vi "RPC Method GreeterService GetFeature.vi"(3 "error in (no error)":errorcluster, 4 "gRPCid in":T1, 5 "DNL_LabVIEW Object in":refnum<class "GreeterServiceImpl.lvclass">) -> (0 "error out":errorcluster, 1 "gRPCid out":T1, 2 "DNL_LabVIEW Object out":refnum<class "GreeterServiceImpl.lvclass">)   [LabVIEW 2019, in "UserCode_impl_server.lvlib" / "GreeterServiceImpl.lvclass"]
uses:
  GreeterServiceImpl.lvclass
  <vilib>/gRPC/LabVIEW gRPC Library/Shared/grpcId.ctl
  Generated_stub_server/RPC Messages/Greeter_res.ctl
  Generated_stub_server/RPC Messages/Greeter_res_res_oneof/Greeter_res_res_oneof.lvclass
  Generated_stub_server/RPC Messages/Greeter_req_req_oneof/Greeter_req_req_oneof.lvclass/Greeter_req_req_oneof.ctl
  Generated_stub_server/RPC Messages/Greeter_res_res_oneof/Greeter_res_res_oneof.lvclass/Greeter_res_res_oneof.ctl
  Generated_stub_server/Generated_stub_server.lvlib
  Generated_stub_server/RPC Messages/Greeter_req_req_oneof/Greeter_req_req_oneof.lvclass
  Generated_stub_server/RPC Service/GreeterServiceStub/GreeterServiceStub.lvclass
  <vilib>/gRPC/LabVIEW gRPC Library/grpc-lvsupport-release.lvlib
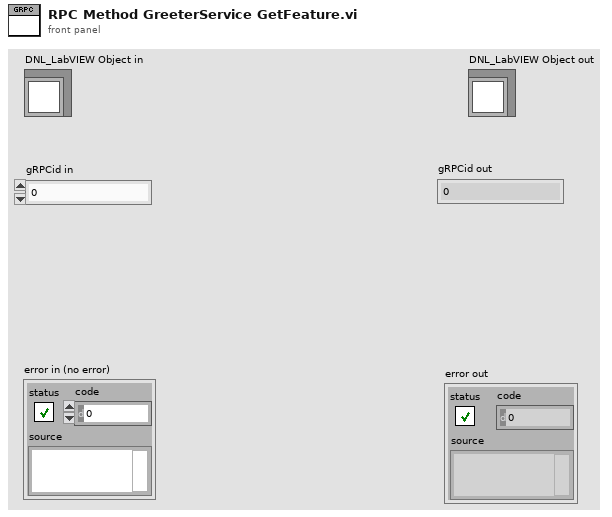
[diagram p1: front panel]
types:
  T1 = typedef "grpc-lvsupport-release.lvlib/grpcId.ctl" = u64
  T2 = typedef "Generated_stub_server.lvlib/Greeter_res.ctl" = cluster{"res_latitude":i32, "Greeter_res_res_oneof":refnum<class "Greeter_res_res_oneof.lvclass">}
  T3 = typedef "Generated_stub_server.lvlib/Greeter_req.ctl" = cluster{"req_latitude":i32, "Greeter_req_req_oneof":refnum<class "Greeter_req_req_oneof.lvclass">}
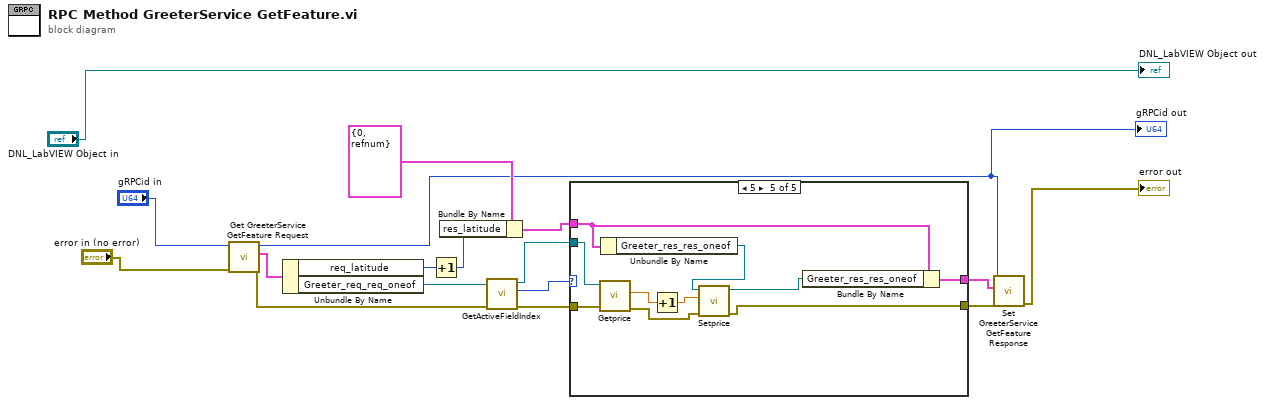
[diagram p0: block diagram]
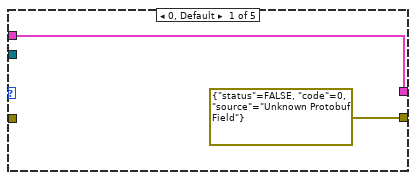
[diagram p2: hidden frame]
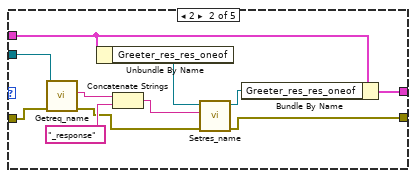
[diagram p3: hidden frame]
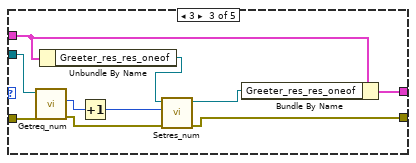
[diagram p4: hidden frame]
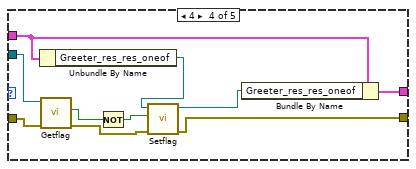
[diagram p5: hidden frame]
diagram:
  n1 = call "Get GreeterService GetFeature Request.vi"("error in (no error)"="error in (no error)", "gRPCid"="gRPCid in") -> ("error out"=w15:errorcluster, "Message Data"=w17:T3, "gRPCid out"=w2:T1)  [unwired: 7 in]
  "gRPCid out" <- w2
  n2 = Unbundle By Name(w17) -> ("req_latitude"=w11:i32, "Greeter_req_req_oneof"=w16:refnum<class "Greeter_req_req_oneof.lvclass">)
  n3 = Increment(x=w11) -> (x+1=w10:i32)
  n4 = Bundle By Name(cluster=T2 {"res_latitude"=0, "Greeter_res_res_oneof"=refnum} ("Greeter_res"), "res_latitude"=w10) -> (w9:T2)
  n5 = call "GetActiveFieldIndex.vi"("error in (no error)"=w15, "OneOfTemplate in"=w16) -> ("error out"=w12:errorcluster, "Active Field Index"=w14:i32, "OneOfTemplate out"=w13:refnum<class "Greeter_req_req_oneof.lvclass">)  [unwired: 7 in]
  n6 = case shown="5" w14 {
    tunnel: w13 -> [_ w30 w38 w48 w59]
    tunnel: w12 -> [_ w29 w37 w47 w58]
    tunnel: w9 -> [w18 w23 w40 w50 w60]
    tunnel: [w18 w21 w39 w49 w52] -> w7
    tunnel: [errorcluster {"status"=FALSE, "code"=0, "source"="Unknown Protobuf Field"} ("error out") w20 w32 w41 w51] -> w8
    frame 0, Default {
    }
    frame 2 {
      n7 = call "Getreq_name.vi"("error in (no error)"=w29, "OneOfTemplate in"=w30) -> ("error out"=w24:errorcluster, "Get_Val"=w28:string)  [unwired: 7 in, 1 out]
      n8 = Unbundle By Name(w23) -> ("Greeter_res_res_oneof"=w26:refnum<class "Greeter_res_res_oneof.lvclass">)
      n9 = Concatenate Strings(w28, "_response" ("string")) -> (w25:string)
      n10 = call "Setres_name.vi"("error in (no error)"=w24, "Set_Val"=w25, "OneOfTemplate in"=w26) -> ("error out"=w20:errorcluster, "OneOfTemplate out"=w22:refnum<class "Greeter_res_res_oneof.lvclass">)  [unwired: 7 in]
      n11 = Bundle By Name(cluster=w23, "Greeter_res_res_oneof"=w22) -> (w21:T2)
    }
    frame 3 {
      n12 = call "Getreq_num.vi"("error in (no error)"=w37, "OneOfTemplate in"=w38) -> ("error out"=w31:errorcluster, "Get_Val"=w36:i32)  [unwired: 7 in, 1 out]
      n13 = Unbundle By Name(w40) -> ("Greeter_res_res_oneof"=w34:refnum<class "Greeter_res_res_oneof.lvclass">)
      n14 = Increment(x=w36) -> (x+1=w35:i32)
      n15 = call "Setres_num.vi"("error in (no error)"=w31, "Set_Val"=w35, "OneOfTemplate in"=w34) -> ("error out"=w32:errorcluster, "OneOfTemplate out"=w33:refnum<class "Greeter_res_res_oneof.lvclass">)  [unwired: 7 in]
      n16 = Bundle By Name(cluster=w40, "Greeter_res_res_oneof"=w33) -> (w39:T2)
    }
    frame 4 {
      n17 = Unbundle By Name(w50) -> ("Greeter_res_res_oneof"=w44:refnum<class "Greeter_res_res_oneof.lvclass">)
      n18 = call "Getflag.vi"("error in (no error)"=w47, "OneOfTemplate in"=w48) -> ("error out"=w43:errorcluster, "Get_Val"=w46:bool)  [unwired: 7 in, 1 out]
      n19 = Not(x=w46) -> (.not. x?=w45:bool)
      n20 = call "Setflag.vi"("error in (no error)"=w43, "Set_Val"=w45, "OneOfTemplate in"=w44) -> ("error out"=w41:errorcluster, "OneOfTemplate out"=w42:refnum<class "Greeter_res_res_oneof.lvclass">)  [unwired: 7 in]
      n21 = Bundle By Name(cluster=w50, "Greeter_res_res_oneof"=w42) -> (w49:T2)
    }
    frame 5 {
      n22 = call "Getprice.vi"("error in (no error)"=w58, "OneOfTemplate in"=w59) -> ("error out"=w54:errorcluster, "Get_Val"=w56:sgl)  [unwired: 7 in, 1 out]
      n23 = Unbundle By Name(w60) -> ("Greeter_res_res_oneof"=w55:refnum<class "Greeter_res_res_oneof.lvclass">)
      n24 = Increment(x=w56) -> (x+1=w57:sgl)
      n25 = call "Setprice.vi"("error in (no error)"=w54, "Set_Val"=w57, "OneOfTemplate in"=w55) -> ("error out"=w51:errorcluster, "OneOfTemplate out"=w53:refnum<class "Greeter_res_res_oneof.lvclass">)  [unwired: 7 in]
      n26 = Bundle By Name(cluster=w60, "Greeter_res_res_oneof"=w53) -> (w52:T2)
    }
  }
  n27 = call "Set GreeterService GetFeature Response.vi"("error in (no error)"=w8, "Message Data"=w7, "gRPCid in"=w2) -> ("error out"=→"error out":errorcluster)  [unwired: 8 in]
  "DNL_LabVIEW Object out" <- "DNL_LabVIEW Object in"
